vi "Add Coin to Cell.vi"(0 "1D Board Array":T1[](array[typedef]), 5 "Cell Index":i32, 7 "Team Number":i32, 11 "error in (no error)":errorcluster) -> (3 "1D Board Array Out":T1[](array[typedef]), 4 "Cell Index":i32, 6 "Win?":bool, 8 "Coins Won":i32, 15 "error out":errorcluster)   [LabVIEW 2014, in "Dragon Tamers.lvlib"]
uses:
  Dragon Tamers.lvlib
  Typedefs/Board Cell.ctl
  Typedefs/Cell Occupancy.ctl
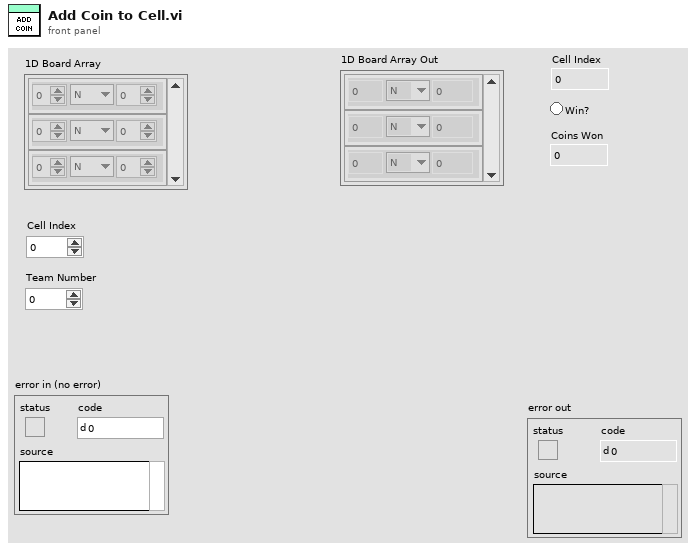
[diagram p1: front panel]
types:
  T1 = typedef "Dragon Tamers.lvlib/Board Cell.ctl" = cluster{"Team":i32, "Occu.":T2, "Count":i32}
  T2 = typedef "Dragon Tamers.lvlib/Cell Occupancy.ctl" = enum16{"N", "C", "K"}
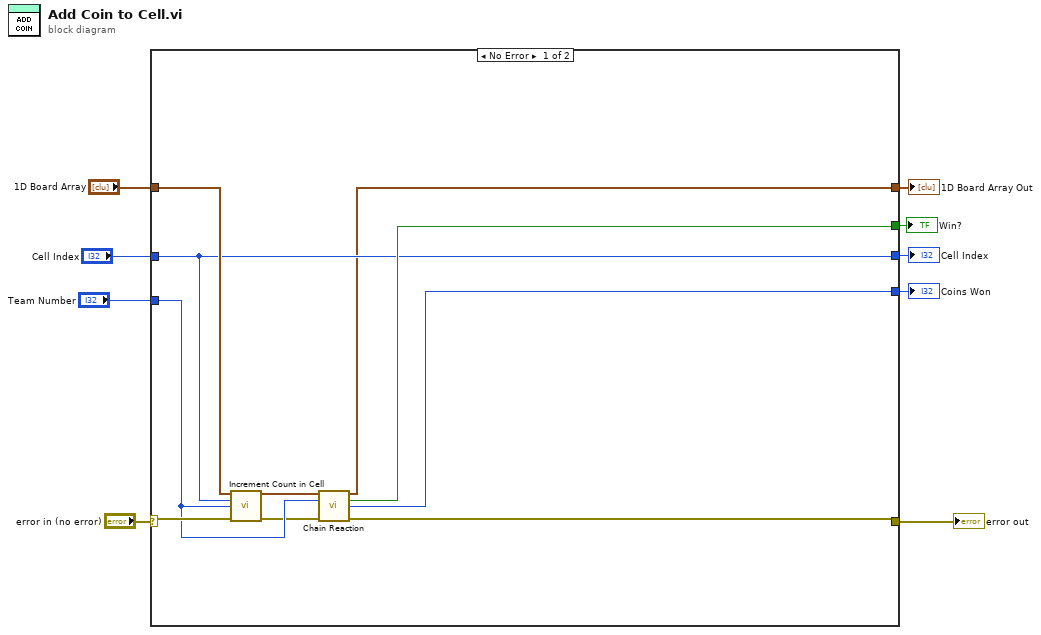
[diagram p0: block diagram]
diagram:
  n1 = case shown="No Error" "error in (no error)" {
    selector: "error in (no error)" -> [w19 w20]
    tunnel: [w14 w20] -> w8
    tunnel: "1D Board Array" -> [w18 _]
    tunnel: "Cell Index" -> [w12 _]
    tunnel: "Team Number" -> [w16 _]
    tunnel: [w13 _] -> w4
    tunnel: [w12 _] -> w3
    tunnel: [w11 _] -> w2
    tunnel: [w10 _] -> w1
    frame No Error {
      n2 = call "Increment Count in Cell.vi"("1D Board"=w18, "Cell Index"=w12, "Team Number"=w16, "error in (no error)"=w19) -> ("1D Board Out"=w17:T1[], "error out"=w15:errorcluster)  [unwired: 9 in, 1 out]
      n3 = call "Chain Reaction.vi"("1D Board"=w17, "Team Number"=w16, "error in (no error)"=w15) -> ("1D Board Out"=w10:T1[], "Won?"=w13:bool, "Coins Won"=w11:i32, "error out"=w14:errorcluster)  [unwired: 9 in]
    }
    frame Error {
    }
  }
  "error out" <- w8
  "Win?" <- w4
  "Cell Index" <- w3
  "Coins Won" <- w2
  "1D Board Array Out" <- w1
